vi "Template Pattern - Caller.vi"(4 "Message Size":T2 {"Message Width" min=-1 step=1; "Message Height" min=-1 step=1}, 6 "Theme":refnum<class "Theme.lvclass">, 7 "standard":T1="info", 8 "error in (no error)":errorcluster, 9 "Graphic":path, 10 "Message":string, 11 "Pop-Up in":refnum<class "Popup.lvclass">) -> (0 "error out":errorcluster, 3 "Pop-Up out":refnum<class "Popup.lvclass">)   [LabVIEW 2021, in "Pop-Up.lvlib" / "Popup.lvclass"]
doc: "<b>Code Developed By:</b>\nDaniel Coons\nTechnology Service Corporation\n1983 S Liberty Drive\nBloomington, IN 47403\nPhone: 812 558-7100\ndaniel.coons@tsc.com\nwww.tsc.com/atcs"
uses:
  Popup.lvclass
  Theme/Theme.lvclass
  message info--typedef.ctl
  Graphics.ctl
  Popup.lvclass/Popup.ctl
  Data Member Access/Read Theme.vi
  Data Member Access/Write Theme.vi
  Pop-Up.lvlib
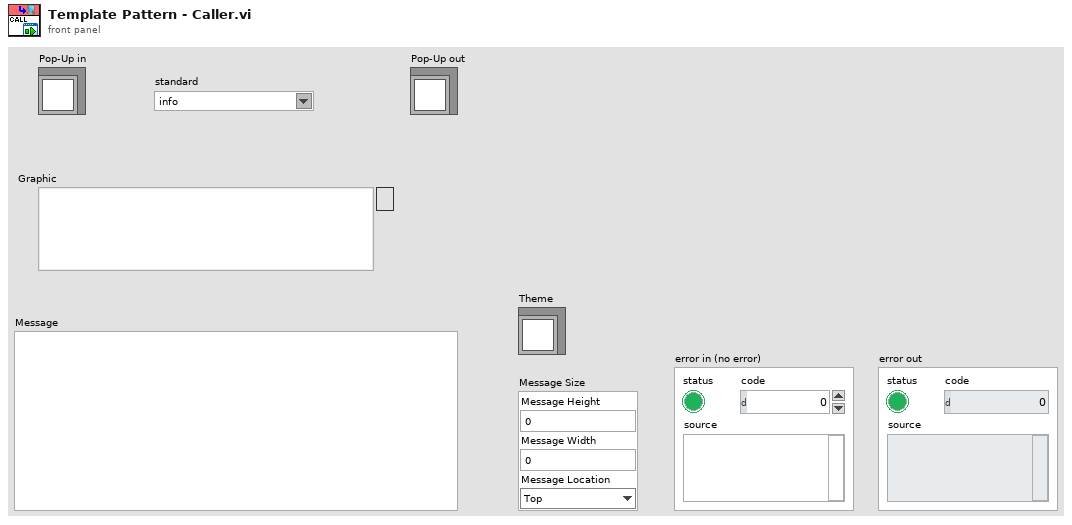
[diagram p1: front panel]
types:
  T1 = typedef "Pop-Up.lvlib/Graphics.ctl" = string
  T2 = typedef "Pop-Up.lvlib/Popup.lvclass/message info--typedef.ctl" = cluster{"Message Height":i32, "Message Width":i32, "Message Location":enum16{"Top", "Bottom", "Right", "Left"}}
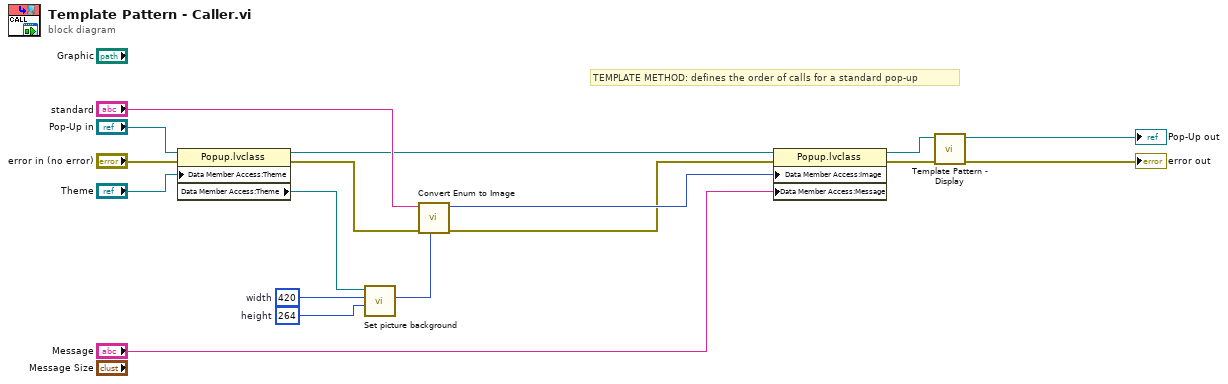
[diagram p0: block diagram]
diagram:
  w4 = i16 264  # height
  w5 = i16 420  # width
  # "TEMPLATE METHOD: defines the order of calls for a standard pop-up"
  n1 = property class="Popup.lvclass"(reference="Pop-Up in", error in="error in (no error)", "Data Member Access:Theme"="Theme") -> (reference out=w1:refnum<class "Popup.lvclass">, error out=w15:errorcluster, "Data Member Access:Theme"=w17:refnum<class "Theme.lvclass">)
  n2 = call "Set picture background.vi"("pic height"=w4, "pic width"=w5, "Theme in"=w17) -> ("background"=w13:picture)  [unwired: 6 in, 2 out]
  n3 = call "Convert Enum to Image.vi"("picture background"=w13, "error in (no error)"=w15, "Graphics"="standard") -> ("error out"=w8:errorcluster, "Image"=w12:picture)  [unwired: 7 in]
  n4 = property class="Popup.lvclass"(reference=w1, error in=w8, "Data Member Access:Image"=w12, "Data Member Access:Message"="Message") -> (reference out=w9:refnum<class "Popup.lvclass">, error out=w6:errorcluster)
  n5 = call "Template Pattern - Display.vi"("error in (no error)"=w6, "PopUp in"=w9) -> ("error out"=→"error out":errorcluster, "PopUp out"=→"Pop-Up out":refnum<class "Popup.lvclass">)  [unwired: 8 in]
